vi "Example.vi"() -> ()   [LabVIEW 2019]
uses:
  Builds/Menu Launcher Module.lvlibp
panel:
  in  "Position":T1(ring)=enum."Bottom Left"
  in  "Stop":bool
  out "Selected Options":string
  in  "Menu File Path":path
  in  "Menu":bool
  # "1. Select Menu File in the menu file path\n2. Run the VI\n3. Select Menu Option to Launch SyncSols Menu\n4. Stop the VI using stop function"
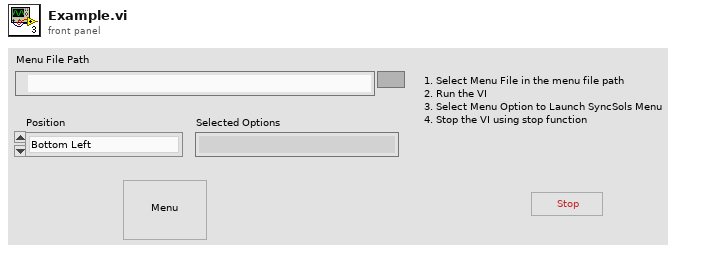
[diagram p1: front panel]
types:
  T1 = enum16{"Top Left", "Top Right", "Bottom Left", "Bottom Right", "Center"}
  T2 = typedef "Menu Launcher Module.lvlibp/Broadcast Events--cluster.ctl" = cluster{"Module Did Init":refnum<user-event>, "Status Updated":refnum<user-event>, "Error Reported":refnum<user-event>, "Module Did Stop":refnum<user-event>, "Update Module Execution Status":refnum<user-event>, "Get Selected Option":refnum<user-event>}
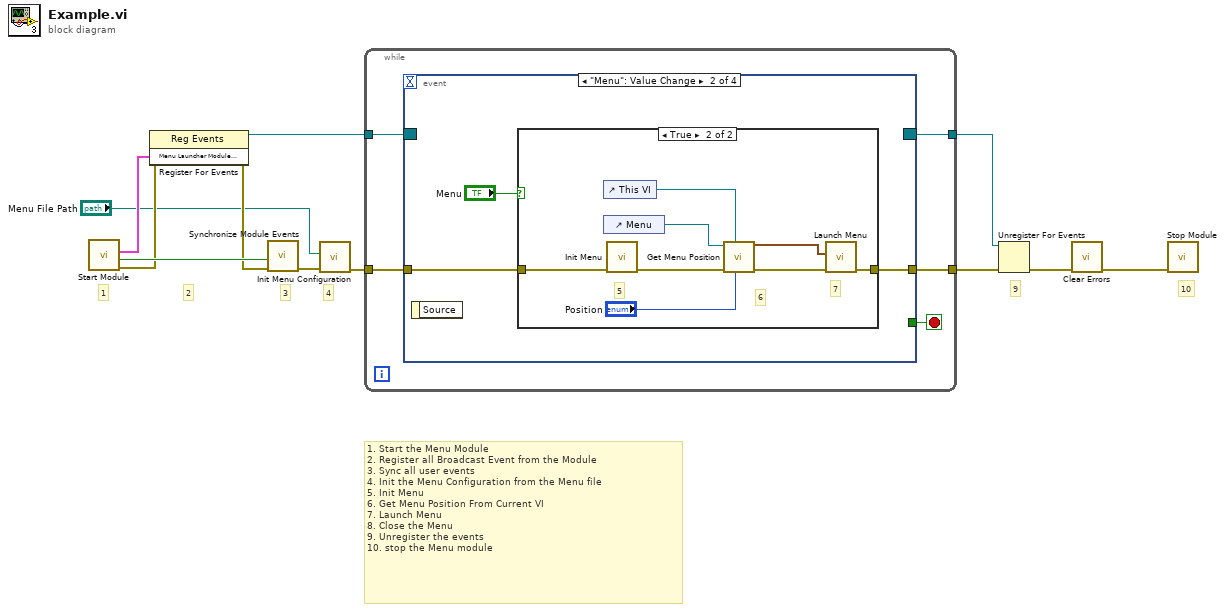
[diagram p0: block diagram]
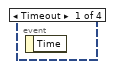
[diagram p2: hidden frame]
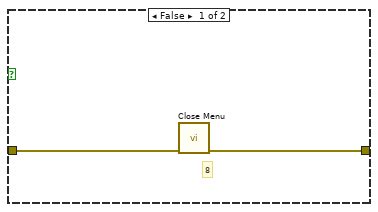
[diagram p3: hidden frame]
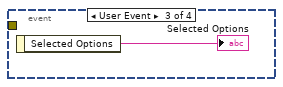
[diagram p4: hidden frame]
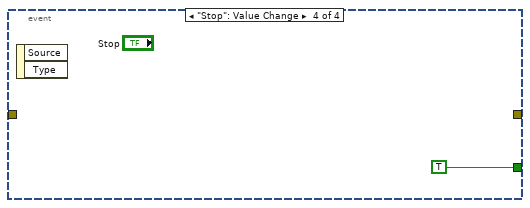
[diagram p5: hidden frame]
diagram:
  # "1. Start the Menu Module\n2. Register all Broadcast Event from the Module\n3. Sync all user events \n4. Init the Menu Configuration from the Menu file\n5. Init Menu\n6. Get Menu Position From Current VI\n7. Launch Menu\n8. Close the Menu\n9. Unregister the events\n10. stop the Menu module"
  # "10"
  # "9"
  # "4"
  # "3"
  # "2"
  # "1"
  n1 = call "Start Module.vi"() -> ("error out"=w9:errorcluster, "Wait for Event Sync?"=w11:bool, "Menu Launcher Module Broadcast Events"=w12:T2)  [unwired: 8 in, 1 out]
  n2 = register-events(error in=w9, w12) -> (reference out=w10:refnum<event-registration>, error out=w8:errorcluster)  [unwired: 1 in]
  n3 = call "Synchronize Module Events.vi"("error in (no error)"=w8, "Wait for Event Sync?"=w11) -> ("error out"=w7:errorcluster)  [unwired: 9 in]
  n4 = call "Init Menu Configuration.vi"("error in (no error)"=w7, "Menu File Path"="Menu File Path") -> ("error out"=w5:errorcluster)  [unwired: 9 in]
  n5 = while {
    tunnel: w10 -> [w17]
    tunnel: w5 -> [w16]
    tunnel: [w15] -> w4
    tunnel: [w14] -> w3
    stop <- w13 stop-if-true
    n6 = event shown="[1] \"Menu\": Value Change" {
      selector: w17 -> [_ _ _ _]
      dyn-events: [_ _ _ _] -> w14
      timeout: _ -> [_ _ _ _]
      tunnel: w16 -> [_ w20 _ _]
      tunnel: [_ w19 _ _] -> w15
      tunnel: [_ _ _ TRUE] -> w13
      event Timeout {
        n7 = event-data() -> ()  [unwired: 1 in, 1 out]
      }
      event "Menu": Value Change {
        n8 = event-data() -> ()  [unwired: 1 in, 1 out]
        n9 = case shown="True" "Menu" {
          tunnel: w20 -> [w22 w30]
          tunnel: [w21 w29] -> w19
          frame False {
            # "8"
            n10 = call "Close Menu.vi"("error in (no error)"=w22) -> ("error out"=w21:errorcluster)  [unwired: 10 in]
          }
          frame True {
            # "6"
            # "7"
            # "5"
            n11 = control-ref of="This VI"() -> (w27:refnum<vi>)
            n12 = control-ref of="Menu"() -> (w28:refnum<vi>)
            n13 = call "Init Menu.vi"("error in (no error)"=w30) -> ("error out"=w26:errorcluster)  [unwired: 10 in]
            n14 = call "Get Menu Position.vi"("Position"="Position", "VI Refnum(Calling VI)"=w27, "error in (no error)"=w26, "Menu Refnum"=w28) -> ("error out"=w25:errorcluster, "Position"=w24:cluster{"Top":i16, "Left":i16})  [unwired: 6 in]
            n15 = call "Launch Menu.vi"("error in (no error)"=w25, "Position"=w24) -> ("error out"=w29:errorcluster)  [unwired: 9 in]
          }
        }
      }
      event User Event {
        n16 = event-data() -> ("Selected Options"=→"Selected Options":string)  [unwired: 1 in]
      }
      event "Stop": Value Change {
        n17 = event-data() -> ()  [unwired: 1 in, 2 out]
      }
    }
  }
  n18 = Unregister For Events(event registration refnum=w3, error in=w4) -> (error out=w2:errorcluster)
  n19 = call <vilib>:"Clear Errors.vi"("error in (no error)"=w2) -> ("error out"=w1:errorcluster)  [unwired: 5 in, 1 out]
  n20 = call "Stop Module.vi"("error in (no error)"=w1) -> ()  [unwired: 10 in, 1 out]
